vi "Main.vi"() -> ()   [LabVIEW 2017]
uses:
  Consumer Message.ctl
  <vilib>/Utility/error.llb/Error Cluster From Error Code.vi
  <vilib>/ErrorRing/Error Ring.xnode
panel:
  in  "Producer Error":bool
  in  "Consumer Error":bool
  out "Consumer Shutdown?":bool
  out "State to Execute":string
  out "High Priority?":bool
  out "Backlog":u8(slide) scale=0.0..100.0
  out "Processed Value":i32
  in  "High Priority Message":bool
  in  "Normal Priority Message":bool
  in  "Stop":bool
  # "Number of enqueued\nmessages waiting to\nbe processed"
  # "Current data being\nprocessed in consumer loop"
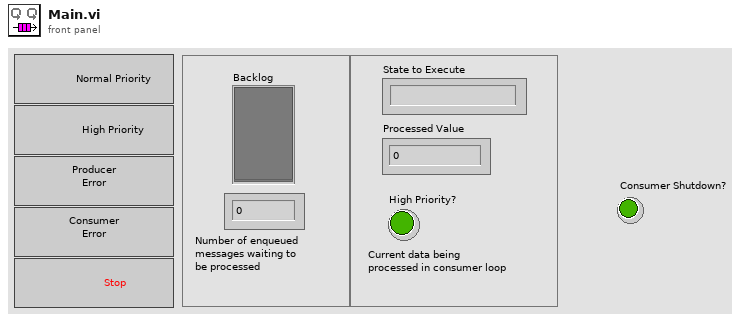
[diagram p1: front panel]
types:
  T1 = typedef "Consumer Message.ctl" = cluster{"Consumer State":string, "Boolean Data":bool, "Numeric Data":i32, "Error":errorcluster}
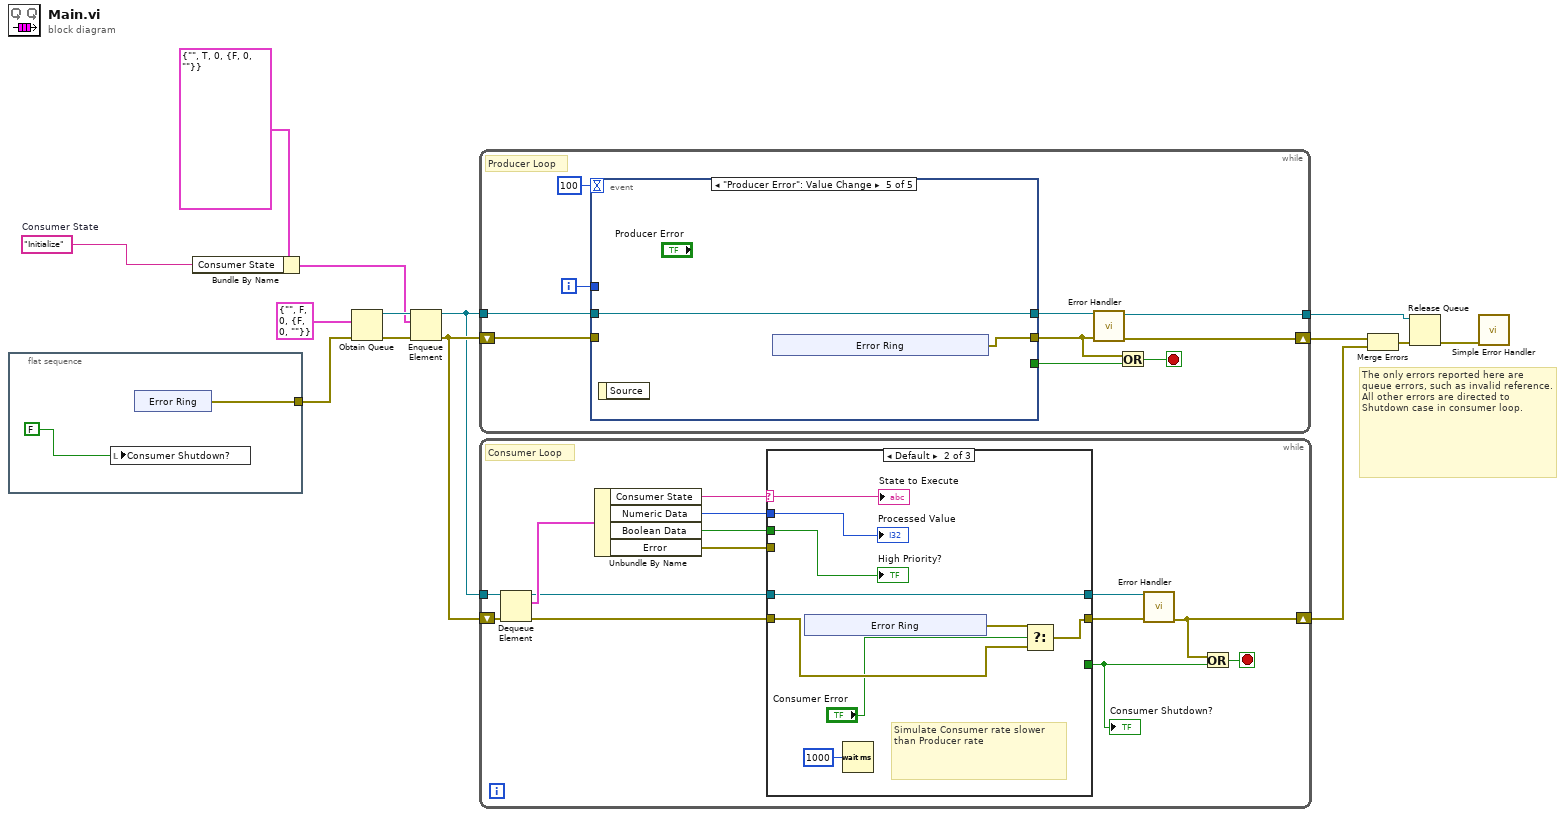
[diagram p0: block diagram]
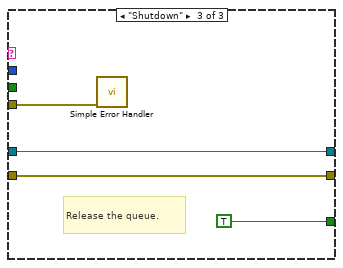
[diagram p3: hidden frame]
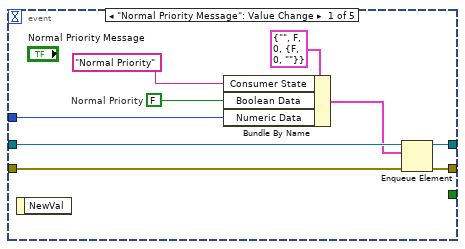
[diagram p4: hidden frame]
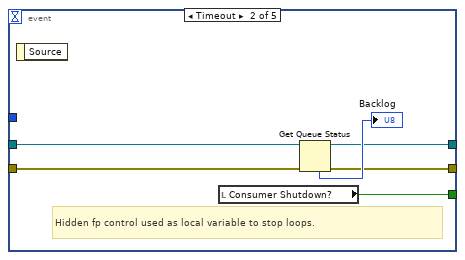
[diagram p5: hidden frame]
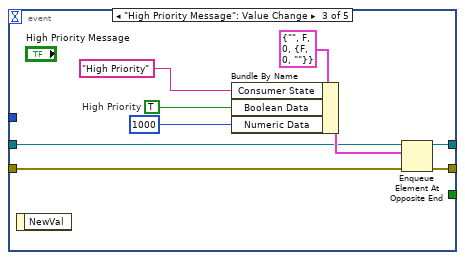
[diagram p6: hidden frame]
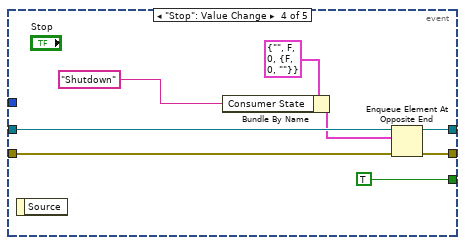
[diagram p7: hidden frame]
diagram:
  w6 = "Initialize"  # Consumer State
  # "The only errors reported here are queue errors, such as invalid reference.  All other errors are directed to Shutdown case in consumer loop."
  n1 = flat-sequence {
    tunnel: [w15] -> w9
    frame #0 {
      n2 = local write "Consumer Shutdown?"(FALSE ("Stop Loops (local)")) -> ()
      n3 = xnode "Error Ring"() -> ("error out"=w15:errorcluster)
    }
  }
  n4 = Bundle By Name(cluster=T1 {"Consumer State"="", "Boolean Data"=TRUE, "Numeric Data"=0, "Error"={"status"=FALSE, "code"=0, "source"=""}} ("Consumer Message"), "Consumer State"=w6) -> (w7:T1)
  n5 = Obtain Queue(element data type=T1 {"Consumer State"="", "Boolean Data"=FALSE, "Numeric Data"=0, "Error"={"status"=FALSE, "code"=0, "source"=""}}, error in (no error)=w9) -> (queue out=w11:refnum<queue>, error out=w14:errorcluster)  [unwired: 3 in, 1 out]
  n6 = Enqueue Element(queue=w11, element=w7, error in (no error)=w14) -> (queue out=w10:refnum<queue>, error out=w12:errorcluster)  [unwired: 1 in, 1 out]
  n7 = while {
    tunnel: w10 -> [w27]
    shift-right: [w19] -> w4
    shift-left: w12 -> [w26]
    tunnel: [w18] -> w1
    i -> [w25]
    stop <- w21 stop-if-true
    # "Producer Loop"
    n8 = event shown="[4] \"Producer Error\": Value Change" {
      selector: _ -> [_ _ _ _ _]
      dyn-events: _ -> [_ _ _ _ _]
      timeout: 100 -> [_ _ _ _ _]
      tunnel: w27 -> [w36 w40 w43 w59 w61]
      tunnel: w26 -> [w34 w39 w50 w57 _]
      tunnel: [w35 w38 w51 w56 w60] -> w20
      tunnel: [_ w42 _ TRUE _] -> w22
      tunnel: w25 -> [w33 _ _ _ _]
      tunnel: [w29 w37 w46 w55 w61] -> w24
      event "Normal Priority Message": Value Change {
        w30 = FALSE  # Normal Priority
        n9 = event-data() -> ()  [unwired: 1 in, 1 out]
        n10 = Bundle By Name(cluster=T1 {"Consumer State"="", "Boolean Data"=FALSE, "Numeric Data"=0, "Error"={"status"=FALSE, "code"=0, "source"=""}}, "Consumer State"="Normal Priority" ("String Data"), "Boolean Data"=w30, "Numeric Data"=w33) -> (w32:T1)
        n11 = Enqueue Element(queue=w36, element=w32, error in (no error)=w34) -> (queue out=w29:refnum<queue>, error out=w35:errorcluster)  [unwired: 1 in, 1 out]
      }
      event Timeout {
        # "Hidden fp control used as local variable to stop loops."
        n12 = event-data() -> ()  [unwired: 1 in, 1 out]
        n13 = local read "Consumer Shutdown?"() -> (w42:bool)
        n14 = Get Queue Status(queue=w40, error in (no error)=w39) -> (queue out=w37:refnum<queue>, error out=w38:errorcluster, # elements in queue=→"Backlog":i32)  [unwired: 1 in, 5 out]
      }
      event "High Priority Message": Value Change {
        w45 = TRUE  # High Priority
        n15 = event-data() -> ()  [unwired: 1 in, 1 out]
        n16 = Bundle By Name(cluster=T1 {"Consumer State"="", "Boolean Data"=FALSE, "Numeric Data"=0, "Error"={"status"=FALSE, "code"=0, "source"=""}}, "Consumer State"="High Priority" ("String Data"), "Boolean Data"=w45, "Numeric Data"=1000) -> (w48:T1)
        n17 = Enqueue Element At Opposite End(queue=w43, element=w48, error in (no error)=w50) -> (queue out=w46:refnum<queue>, error out=w51:errorcluster)  [unwired: 1 in, 1 out]
      }
      event "Stop": Value Change {
        n18 = event-data() -> ()  [unwired: 1 in, 1 out]
        n19 = Bundle By Name(cluster=T1 {"Consumer State"="", "Boolean Data"=FALSE, "Numeric Data"=0, "Error"={"status"=FALSE, "code"=0, "source"=""}}, "Consumer State"="Shutdown") -> (w52:T1)
        n20 = Enqueue Element At Opposite End(queue=w59, element=w52, error in (no error)=w57) -> (queue out=w55:refnum<queue>, error out=w56:errorcluster)  [unwired: 1 in, 1 out]
      }
      event "Producer Error": Value Change {
        n21 = event-data() -> ()  [unwired: 1 in, 1 out]
        n22 = xnode "Error Ring"() -> ("error out"=w60:errorcluster)
      }
    }
    n23 = call "Error Handler.vi"("error in"=w20, "queue in"=w24) -> ("error out"=w19:errorcluster, "queue out"=w18:refnum<queue>)  [unwired: 8 in]
    n24 = Or(x=w20, y=w22) -> (x .or. y?=w21:bool)
  }
  n25 = while {
    tunnel: w10 -> [w79]
    shift-right: [w68] -> w5
    shift-left: w12 -> [w78]
    stop <- w69 stop-if-true
    # "Consumer Loop"
    n26 = Dequeue Element(queue=w79, error in (no error)=w78) -> (queue out=w67:refnum<queue>, element=w77:T1, error out=w66:errorcluster)  [unwired: 1 in, 1 out]
    n27 = Unbundle By Name(w77) -> ("Consumer State"=w76:string, "Numeric Data"=w75:i32, "Boolean Data"=w74:bool, "Error"=w71:errorcluster)
    n28 = case shown="Default" w76 {
      selector: w76 -> [_ w87 _]
      tunnel: [_ _ TRUE] -> w70
      tunnel: w66 -> [w80 w85 w96]
      tunnel: [w80 w82 w96] -> w73
      tunnel: w75 -> [_ w90 _]
      tunnel: w74 -> [_ w89 _]
      tunnel: w67 -> [w81 w88 w97]
      tunnel: [w81 w88 w97] -> w72
      tunnel: w71 -> [_ _ w98]
      frame "Initialize" {
      }
      frame Default {
        # "Simulate Consumer rate slower than Producer rate"
        n29 = xnode "Error Ring"() -> ("error out"=w83:errorcluster)
        n30 = Wait (ms)(milliseconds to wait=u32 1000) -> ()  [unwired: 1 out]
        n31 = Select(t=w83, s="Consumer Error", f=w85) -> (s? t:f=w82:errorcluster)
        "Processed Value" <- w90
        "High Priority?" <- w89
        "State to Execute" <- w87
      }
      frame "Shutdown" {
        # "Release the queue."
        n32 = call <vilib>:"Simple Error Handler.vi"("error in (no error)"=w98) -> ()  [unwired: 4 in, 5 out]
      }
    }
    "Consumer Shutdown?" <- w70
    n33 = call "Error Handler.vi"("error in"=w73, "queue in"=w72) -> ("error out"=w68:errorcluster)  [unwired: 8 in, 1 out]
    n34 = Or(x=w68, y=w70) -> (x .or. y?=w69:bool)
  }
  n35 = Merge Errors(w4, w5) -> (w3:errorcluster)
  n36 = Release Queue(queue=w1, error in (no error)=w3) -> (error out=w2:errorcluster)  [unwired: 1 in, 2 out]
  n37 = call <vilib>:"Simple Error Handler.vi"("error in (no error)"=w2) -> ()  [unwired: 4 in, 5 out]
